vi "Sign Test (paired samples).vi"(6 "alternative hypothesis":i32(ring) items=["median(x) != median(y)"=0, "median(x) > median(y)"=1, "median(x) < median(y)"=-1], 9 "significance level":dbl=0.05, 10 "sample set y":dbl[](array[numeric]), 11 "sample set x":dbl[](array[numeric])) -> (0 "error":i32, 2 "p value":dbl=0.05 format="%.6g", 3 "reject null hypothesis":bool)   [LabVIEW 2020, in "NI_Gmath.lvlib"]
doc: "Tests hypotheses about the <B>median</B> of continuous distributions. You must manually select the polymorphic instance to use."
uses:
  <vilib>/gmath/NI_Gmath.lvlib
panel:
  # "Sign Test"
  # "null hypothesis\nmedian(pop) = median"
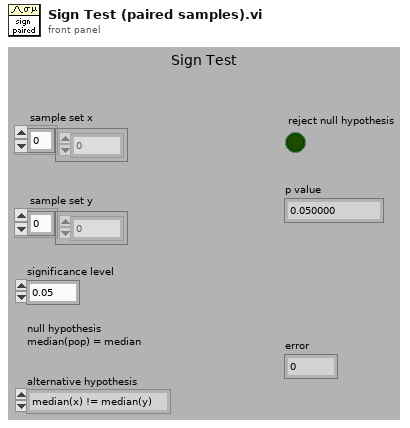
[diagram p1: front panel]
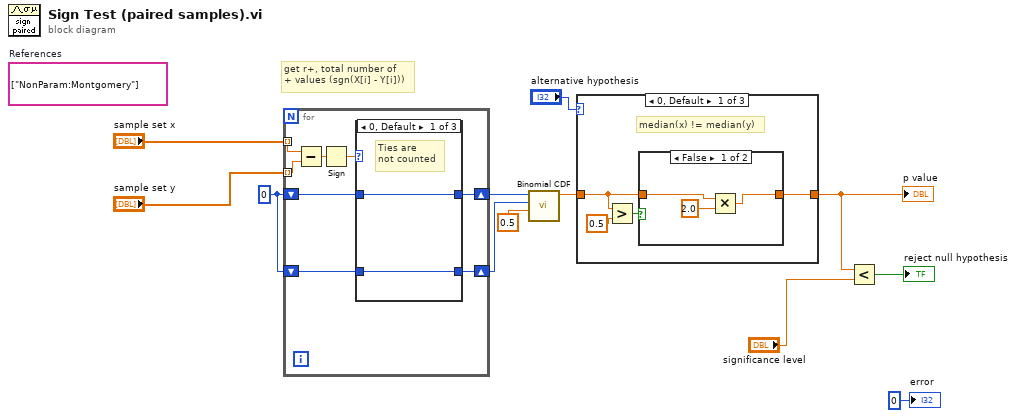
[diagram p0: block diagram]
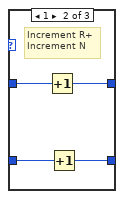
[diagram p2: hidden frame]
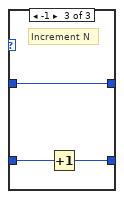
[diagram p3: hidden frame]
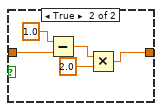
[diagram p4: hidden frame]
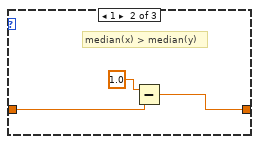
[diagram p5: hidden frame]
diagram:
  (unwired) string[] ["NonParam:Montgomery"]  # References
  w2 = 0
  # "get r+, total number of\n+ values (sgn(X[i] - Y[i]))"
  n1 = for {
    tunnel: "sample set x" -> [w19] mode=indexing
    tunnel: "sample set y" -> [w20] mode=indexing
    shift-right: [w13] -> w6
    shift-left: w2 -> [w14]
    shift-right: [w15] -> w1
    shift-left: w2 -> [w16]
    n2 = Subtract(x=w19, y=w20) -> (x-y=w18:dbl)
    n3 = Sign(1:w18) -> (0:w17:dbl)
    n4 = case shown="0, Default" w17 {
      tunnel: w16 -> [w22 w24 w29]
      tunnel: [w22 w23 w28] -> w15
      tunnel: w14 -> [w21 w26 w27]
      tunnel: [w21 w25 w27] -> w13
      frame 0, Default {
        # "Ties are\nnot counted"
      }
      frame 1 {
        # "Increment R+\nIncrement N"
        n5 = Increment(x=w26) -> (x+1=w25:i32)
        n6 = Increment(x=w24) -> (x+1=w23:i32)
      }
      frame -1 {
        # "Increment N"
        n7 = Increment(x=w29) -> (x+1=w28:i32)
      }
    }
  }
  n8 = call <vilib>:"Binomial CDF.vi"("p"=0.5 ("a"), "n"=w1, "x"=w6) -> ("cdf(x)"=w4:dbl)  [unwired: 7 in, 1 out]
  n9 = case shown="0, Default" "alternative hypothesis" {
    tunnel: [w33 w43 w45] -> w9
    tunnel: w4 -> [w32 w42 w45]
    frame 0, Default {
      # "median(x) != median(y)"
      n10 = Greater?(x=w32, y=0.5) -> (0:w30:bool)
      n11 = case shown="False" w30 {
        tunnel: [w34 w38] -> w33
        tunnel: w32 -> [w35 w37]
        frame False {
          n12 = Multiply(x=w35, y=2.0) -> (x*y=w34:dbl)
        }
        frame True {
          n13 = Subtract(x=1.0, y=w37) -> (x-y=w39:dbl)
          n14 = Multiply(x=w39, y=2.0) -> (x*y=w38:dbl)
        }
      }
    }
    frame 1 {
      # "median(x) > median(y)"
      n15 = Subtract(x=1.0, y=w42) -> (x-y=w43:dbl)
    }
    frame -1 {
      # "median(x) < median(y)"
    }
  }
  "p value" <- w9
  n16 = Less?(x=w9, y="significance level") -> (x < y?=→"reject null hypothesis":bool)
  "error" <- 0 ("error")
